vi "VisionTracking Y.vi"(1 "Robot Mode":T1, 2 "Tweak":dbl) -> (0 "output":dbl)   [LabVIEW 2012]
uses:
  <vilib>/Rock Robotics/WPI/DriverStation/WPI_DriverStationRobotMode.ctl
  typedefs/fg_typedef.ctl
  <vilib>/addons/control/pid/pid.llb/PID (DBL).vi
  <vilib>/addons/control/pid/NI_PID_pid.lvlib
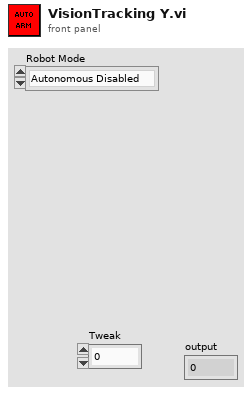
[diagram p1: front panel]
types:
  T1 = typedef "WPI_DriverStationRobotMode.ctl" = enum16{"Autonomous Disabled", "Autonomous Enabled", "Teleop Disabled", "Teleop Enabled", "Timeout", "Finish"}
  T2 = cluster{"Left":dbl, "Top":dbl, "Right":dbl, "Bottom":dbl, "Target CoM X":dbl, "Target CoM Y":dbl}
  T3 = typedef "fg_typedef.ctl" = enum16{"Get", "Set"}
  T4 = cluster{"Left":bool, "Top":bool, "Right":bool, "Bottom":bool, "Target CoM X":bool, "Target CoM Y":bool}
  T5 = typedef "WPI_CameraDevRef.ctl" = cluster{"Camera Address":string, "CameraStatus":errorcluster, "Acquire Image Notifier":refnum<notifier>}
  T6 = typedef "WPI_EncoderDevRef.ctl" = cluster{"DevStatus":errorcluster, "EncoderIndex":T7, "CounterIndex":T8, "DistancePerCount":dbl, "Decoding Type":T9}
  T7 = typedef "FPGA_EncoderIdx.ctl" = enum8{"Enc 0", "Enc 1", "Enc 2", "Enc 3", "Invalid"}
  T8 = typedef "FPGA_CounterCtrSystemIndex.ctl" = enum8{"Ctr 0", "Ctr 1", "Ctr 2", "Ctr 3", "Ctr 4", "Ctr 5", "Ctr 6", "Ctr 7", "Invalid"}
  T9 = typedef "WPI_EncoderType.ctl" = enum16{"1x", "2x", "4x"}
  T10 = typedef "WPI_CameraImageSize.ctl" = enum16{"640x480", "320x240", "160x120"}
  T11 = cluster{"proportional gain (Kc)":dbl, "integral time (Ti, min)":dbl, "derivative time (Td, min)":dbl}
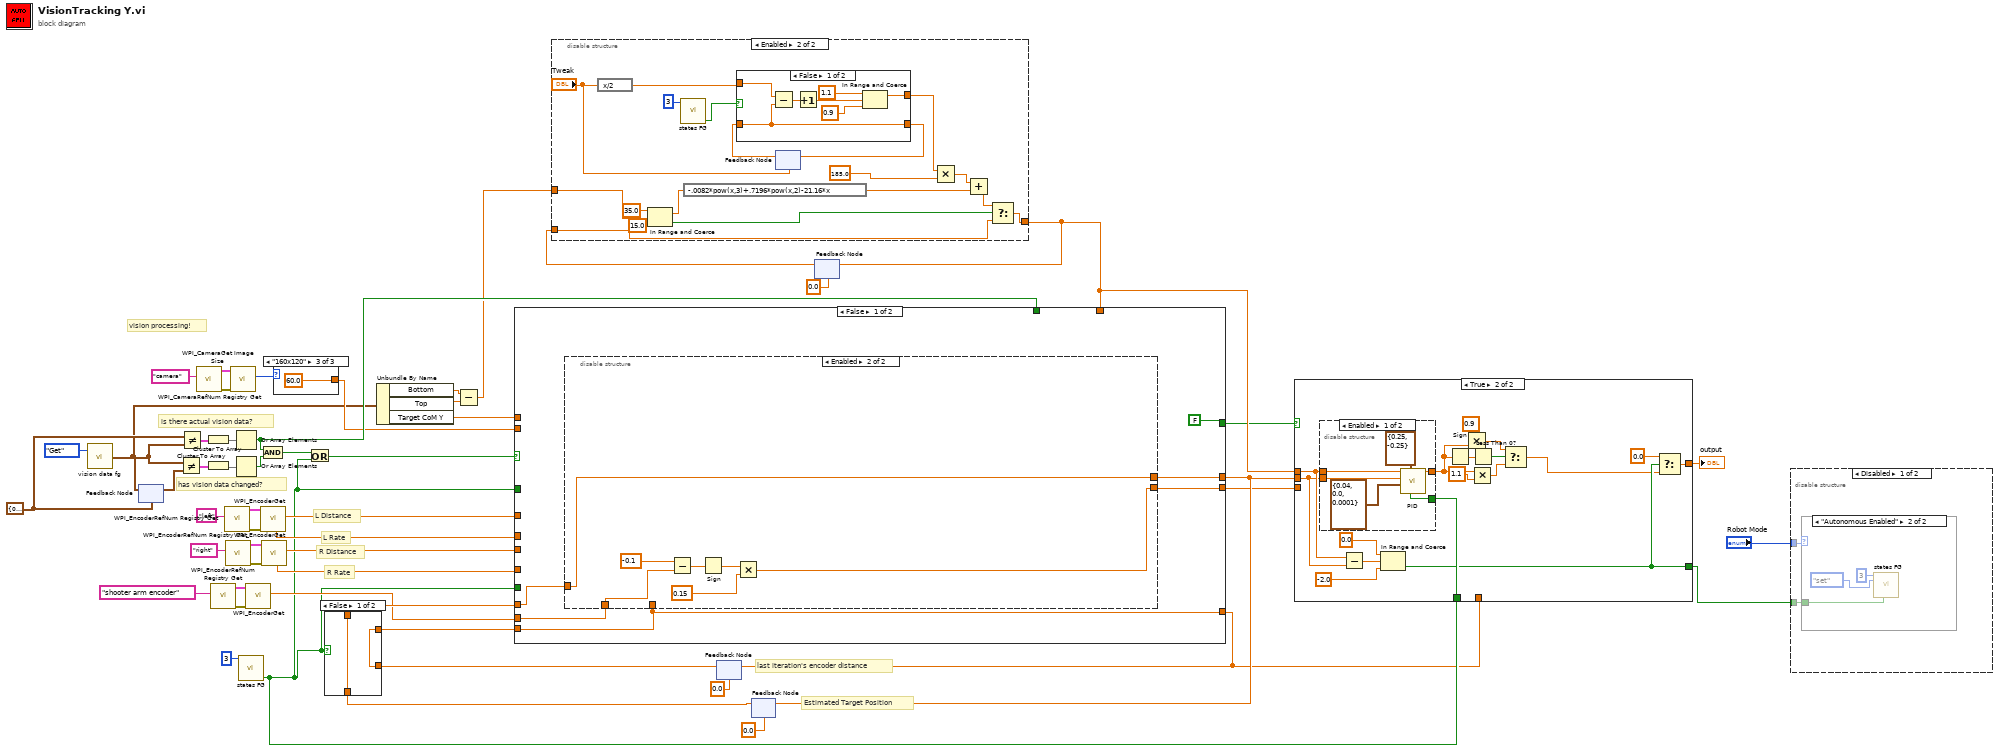
[diagram p0: block diagram]
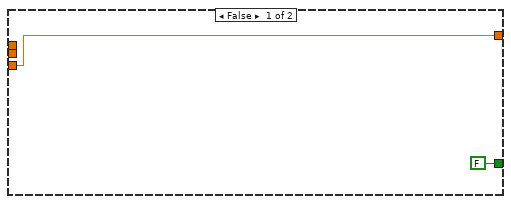
[diagram p4: hidden frame]
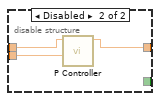
[diagram p5: hidden frame]
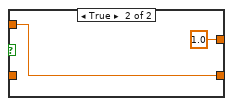
[diagram p7: hidden frame]
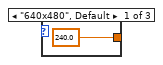
[diagram p8: hidden frame]
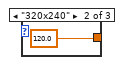
[diagram p9: hidden frame]
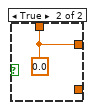
[diagram p10: hidden frame]
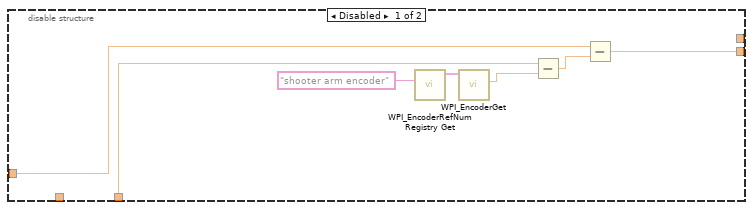
[diagram p11: hidden frame]
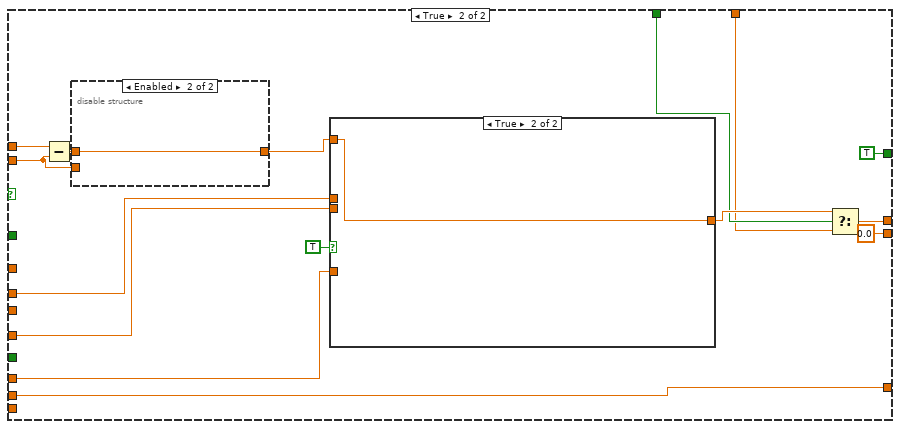
[diagram p12: hidden frame]
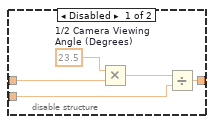
[diagram p13: hidden frame]
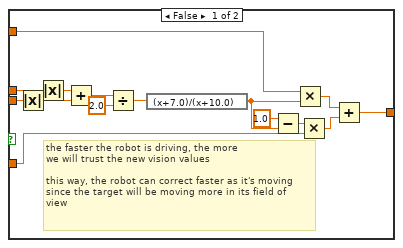
[diagram p14: hidden frame]
diagram:
  w26 = T2 {"Left"=0.0, "Top"=0.0, "Right"=0.0, "Bottom"=0.0, "Target CoM X"=0.0, "Target CoM Y"=0.0} ("Input")
  # "Estimated Target Position"
  # "last iteration's encoder distance"
  # "R Distance"
  # "R Rate"
  # "L Distance"
  # "L Rate"
  # "has vision data changed?"
  # "is there actual vision data?"
  # "vision processing!"
  n1 = call "vision data fg.vi"("Menu"=fg_typedef."Get") -> ("Output"=w20:T2)  [unwired: 1 in]
  n2 = feedback #1(w26) -> (w45:T2)
  n3 = feedback-in #1(w20) -> ()
  n4 = Not Equal?(x=w20, y=w45) -> (x != y?=w50:T4)
  n5 = Not Equal?(x=w26, y=w20) -> (x != y?=w49:T4)
  n6 = call <vilib>:"WPI_CameraRefNum Registry Get.vi"("refnum name"="camera") -> ("error out"=w24:errorcluster, "CameraDevRef"=w23:T5)  [unwired: 9 in]
  n7 = Cluster To Array(cluster=w49) -> (array=w46:bool[])
  n8 = Cluster To Array(cluster=w50) -> (array=w47:bool[])
  n9 = call <vilib>:"WPI_EncoderRefNum Registry Get.vi"("refnum name"="shooter arm encoder") -> ("error out"=w10:errorcluster, "EncoderDevRef"=w11:T6)  [unwired: 9 in]
  n10 = call <vilib>:"WPI_EncoderRefNum Registry Get.vi"("refnum name"="left") -> ("error out"=w40:errorcluster, "EncoderDevRef"=w41:T6)  [unwired: 9 in]
  n11 = call <vilib>:"WPI_EncoderRefNum Registry Get.vi"("refnum name"="right") -> ("error out"=w38:errorcluster, "EncoderDevRef"=w39:T6)  [unwired: 9 in]
  n12 = call <vilib>:"WPI_CameraGet Image Size.vi"("error in (no error)"=w24, "CameraDevRef"=w23) -> ("Image Size"=w22:T10)  [unwired: 7 in, 2 out]
  n13 = Or Array Elements(Boolean array=w46) -> (logical OR=w27:bool)
  n14 = Or Array Elements(Boolean array=w47) -> (logical OR=w48:bool)
  n15 = call "states FG.vi"("Loop ID"=3) -> ("first call?"=w5:bool)  [unwired: 7 in, 3 out]
  n16 = call <vilib>:"WPI_EncoderGet.vi"("error in (no error)"=w10, "EncoderDevRef"=w11) -> ("Distance"=w8:dbl)  [unwired: 4 in, 5 out]
  n17 = And(x=w27, y=w48) -> (x .and. y?=w51:bool)
  n18 = call <vilib>:"WPI_EncoderGet.vi"("error in (no error)"=w40, "EncoderDevRef"=w41) -> ("Distance"=w37:dbl, "Rate"=w36:dbl)  [unwired: 4 in, 4 out]
  n19 = call <vilib>:"WPI_EncoderGet.vi"("error in (no error)"=w38, "EncoderDevRef"=w39) -> ("Distance"=w35:dbl, "Rate"=w34:dbl)  [unwired: 4 in, 4 out]
  n20 = case shown="\"160x120\"" w22 {
    tunnel: [240.0 120.0 60.0] -> w21
    frame "640x480", Default {
    }
    frame "320x240" {
    }
    frame "160x120" {
    }
  }
  n21 = Or(x=w51, y=w5) -> (x .or. y?=w43:bool)
  n22 = Unbundle By Name(w20) -> ("Bottom"=w19:dbl, "Top"=w18:dbl, "Target CoM Y"=w13:dbl)
  n23 = Subtract(x=w19, y=w18) -> (x-y=w12:dbl)
  n24 = feedback #2(0.0) -> (w29:dbl)
  n25 = feedback #3(0.0) -> (w28:dbl)
  n26 = case shown="False" w5 {
    tunnel: [w57 w59] -> w32
    tunnel: [w58 w59] -> w30
    tunnel: w29 -> [w58 _]
    tunnel: w28 -> [w57 _]
    frame False {
    }
    frame True {
      w59 = 0.0
    }
  }
  n27 = feedback #4(0.0) -> (w15:dbl)
  n28 = disable-structure shown="Enabled" {
    disable-tunnel: [_ w73] -> w16
    disable-tunnel: w12 -> [_ w75]
    disable-tunnel: w15 -> [_ w70]
    frame Disabled {
    }
    frame Enabled {
      n29 = expression code="x/2"("Tweak") -> (w60:dbl)
      n30 = In Range and Coerce(upper limit=35.0, x=w75, lower limit=15.0) -> (coerced(x)=w74:dbl, In Range?=w71:bool)
      n31 = call "states FG.vi"("Loop ID"=3) -> ("first call?"=w66:bool)  [unwired: 7 in, 3 out]
      n32 = expression code="-.0082*pow(x,3)+.7196*pow(x,2)-21.16*x"(w74) -> (w72:dbl)
      n33 = feedback #5("Tweak") -> (w64:dbl)
      n34 = case shown="False" w66 {
        tunnel: w60 -> [w84 w86]
        tunnel: [w83 w86] -> w65
        tunnel: w64 -> [w83 _]
        tunnel: [w80 1.0 ("upper limit")] -> w62
        frame False {
          n35 = Subtract(x=w84, y=w83) -> (x-y=w79:dbl)
          n36 = Increment(x=w79) -> (x+1=w78:dbl)
          n37 = In Range and Coerce(upper limit=1.1, x=w78, lower limit=0.9) -> (coerced(x)=w80:dbl)  [unwired: 1 out]
        }
        frame True {
        }
      }
      n38 = feedback-in #5(w65) -> ()
      n39 = Multiply(x=w62, y=185.0 ("y ofset")) -> (x*y=w63:dbl)
      n40 = Add(x=w63, y=w72) -> (x+y=w69:dbl)
      n41 = Select(t=w69, s=w71, f=w70) -> (s? t:f=w73:dbl)
    }
  }
  n42 = case shown="False" w43 {
    tunnel: w37 -> [_ _]
    tunnel: w36 -> [_ w121]
    tunnel: w35 -> [_ _]
    tunnel: w34 -> [_ w120]
    tunnel: w5 -> [_ _]
    tunnel: w32 -> [w91 w119]
    tunnel: [w87 w118] -> w17
    tunnel: w30 -> [w92 _]
    tunnel: [w92 w109] -> w3
    tunnel: w16 -> [_ w115]
    tunnel: w27 -> [_ w116]
    tunnel: w5 -> [_ _]
    tunnel: w21 -> [_ w114]
    tunnel: w13 -> [_ w111]
    tunnel: w8 -> [w90 w109]
    tunnel: [FALSE TRUE] -> w7
    tunnel: [w88 0.0] -> w6
    frame False {
      n43 = disable-structure shown="Enabled" {
        disable-tunnel: w92 -> [w97 _]
        disable-tunnel: w91 -> [w94 w100]
        disable-tunnel: [w93 w101] -> w88
        disable-tunnel: w90 -> [_ w105]
        disable-tunnel: [_ w100] -> w87
        frame Disabled {
          n44 = call <vilib>:"WPI_EncoderRefNum Registry Get.vi"("refnum name"="shooter arm encoder") -> ("EncoderDevRef"=w99:T6)  [unwired: 9 in, 1 out]
          n45 = call <vilib>:"WPI_EncoderGet.vi"("EncoderDevRef"=w99) -> ("Distance"=w96:dbl)  [unwired: 5 in, 5 out]
          n46 = Subtract(x=w97, y=w96) -> (x-y=w95:dbl)
          n47 = Subtract(x=w94, y=w95) -> (x-y=w93:dbl)
        }
        frame Enabled {
          n48 = Subtract(x=-0.1, y=w105) -> (x-y=w104:dbl)
          n49 = Sign(1:w104) -> (0:w103:dbl)
          n50 = Multiply(x=w103, y=0.15 ("speed")) -> (x*y=w101:dbl)
        }
      }
    }
    frame True {
      n51 = Subtract(x=w111, y=w114) -> (x-y=w112:dbl)
      n52 = disable-structure shown="Enabled" {
        disable-tunnel: w114 -> [w124 _]
        disable-tunnel: [w123 w127] -> w113
        disable-tunnel: w112 -> [w122 w127]
        frame Disabled {
          w126 = 23.5  # 1/2 Camera Viewing Angle (Degrees)
          n53 = Multiply(x=w126, y=w122) -> (x*y=w125:dbl)
          n54 = Divide(x=w125, y=w124) -> (x/y=w123:dbl)
        }
        frame Enabled {
        }
      }
      n55 = case shown="True" TRUE {
        tunnel: w121 -> [w138 _]
        tunnel: w120 -> [w137 _]
        tunnel: w113 -> [w130 w143]
        tunnel: [w129 w143] -> w117
        tunnel: w119 -> [w128 _]
        frame False {
          # "the faster the robot is driving, the more\nwe will trust the new vision values\n\nthis way, the robot can correct faster as it's moving\nsince the target will be moving more in its field of\nview"
          n56 = Absolute Value(x=w137) -> (abs(x)=w142:dbl)
          n57 = Absolute Value(x=w138) -> (abs(x)=w141:dbl)
          n58 = Add(x=w141, y=w142) -> (x+y=w139:dbl)
          n59 = Divide(x=w139, y=2.0) -> (x/y=w136:dbl)
          n60 = expression code="(x+7.0)/(x+10.0)"(w136) -> (w131:dbl)
          n61 = Subtract(x=1.0, y=w131) -> (x-y=w134:dbl)
          n62 = Multiply(x=w130, y=w131) -> (x*y=w132:dbl)
          n63 = Multiply(x=w134, y=w128) -> (x*y=w133:dbl)
          n64 = Add(x=w132, y=w133) -> (x+y=w129:dbl)
        }
        frame True {
        }
      }
      n65 = Select(t=w117, s=w116, f=w115) -> (s? t:f=w118:dbl)
    }
  }
  n66 = feedback-in #2(w3) -> ()
  n67 = feedback-in #3(w17) -> ()
  n68 = feedback-in #4(w16) -> ()
  n69 = case shown="True" w7 {
    tunnel: [w145 w162] -> w4
    tunnel: w17 -> [_ w159]
    tunnel: w16 -> [_ w160]
    tunnel: w6 -> [w145 _]
    tunnel: w5 -> [_ w155]
    tunnel: w3 -> [_ _]
    tunnel: [FALSE w147] -> w2
    frame False {
    }
    frame True {
      n70 = disable-structure shown="Enabled" {
        disable-tunnel: [w167 w169] -> w152
        disable-tunnel: w159 -> [w166 w170]
        disable-tunnel: w160 -> [w165 w171]
        disable-tunnel: w155 -> [w164 _]
        frame Enabled {
          n71 = call-poly <vilib>:"PID.vi"("reinitialize? (F)"=w164, "output range"=cluster{"output high":dbl, "output low":dbl} {"output high"=0.25, "output low"=-0.25}, "PID gains"=T11 {"proportional gain (Kc)"=0.04, "integral time (Ti, min)"=0.0, "derivative time (Td, min)"=0.0001}, "process variable"=w166, "setpoint"=w165) -> ("output"=w167:dbl)  [unwired: 5 in, 1 out]
        }
        frame Disabled {
          n72 = call "P Controller.vi"("Setpoint"=w171, "Process Variable"=w170) -> ("Output"=w169:dbl)  [unwired: 6 in]
        }
      }
      n73 = Subtract(x=w160, y=w159) -> (x-y=w158:dbl)
      n74 = In Range and Coerce(upper limit=0.0, x=w158, lower limit=-2.0) -> (In Range?=w147:bool)  [unwired: 1 out]
      n75 = Sign(1:w152) -> (0:w154:dbl)
      n76 = Multiply(x=0.9 ("down"), y=w152) -> (x*y=w151:dbl)
      n77 = Multiply(x=w152, y=1.1 ("up")) -> (x*y=w149:dbl)
      n78 = Less Than 0?(x=w154) -> (x < 0?=w153:bool)
      n79 = Select(t=w151, s=w153, f=w149) -> (s? t:f=w146:dbl)
      n80 = Select(t=0.0, s=w147, f=w146) -> (s? t:f=w162:dbl)
    }
  }
  "output" <- w4
  n81 = disable-structure shown="Disabled" {
    disable-tunnel: w2 -> [w173 _]
    disable-tunnel: "Robot Mode" -> [w172 _]
    frame Disabled {
      n82 = case shown="\"Autonomous Enabled\"" w172 {
        tunnel: w173 -> [_ w174]
        frame "Autonomous Disabled", Default {
        }
        frame "Autonomous Enabled" {
          n83 = call "states FG.vi"("exit in"=w174, "menu (get)"=enum16{"set", "get"}."set", "Loop ID"=3) -> ()  [unwired: 5 in, 4 out]
        }
      }
    }
    frame Enabled {
    }
  }
